vi "GetDefaultParams.vi"(8 "error in (no error)":errorcluster, 10 "Path":path, 11 "StandardFunction in":refnum<class "StandardFunction.lvclass">) -> (0 "error out":errorcluster, 3 "StandardFunction out":refnum<class "StandardFunction.lvclass">)   [LabVIEW 2018, in "Functions.lvlib" / "StandardFunction.lvclass"]
uses:
  StandardFunction.lvclass
  X:/Projects/NistPluggableModules/dev/NistPluggableModules/FGen/MemberClasses/FunctionBaseClass/FunctionBase.lvclass
  TypeDefs/StdWfrms.ctl
  TypeDefs/StdWfrm.ctl
  FunctionBaseClass/FunctionBase.lvclass/FunctionBase.ctl
  StandardFunction.lvclass/StandardFunction.ctl
  FunctionBaseClass/Accessors/Read FunctionIniFilePath.vi
  Accessors/Write StandardWfrms.vi
  FunctionBaseClass/FunctionBase.lvclass
  <vilib>/Utility/config.llb/NI_LVConfig.lvlib
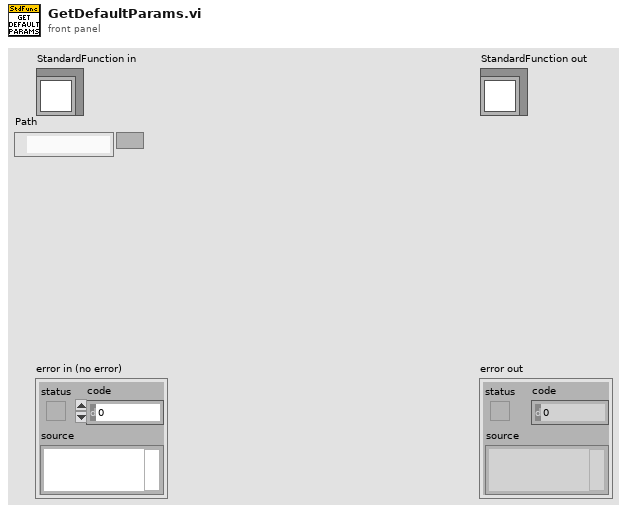
[diagram p1: front panel]
types:
  T1 = typedef "Functions.lvlib/StandardFunction.lvclass/StdWfrms.ctl" = cluster{"Count":u16, "StandardWfrm":T2[]}
  T2 = typedef "Functions.lvlib/StandardFunction.lvclass/StdWfrm.ctl" = cluster{"Amplitude":dbl, "DcOffset":dbl, "DutyCycle":dbl, "Frequency":dbl, "Phase":dbl, "Waveform":enum16{"Sine", "Square", "Triangle", "Ramp Up", "Ramp Down", "DC"}, "Handle":string}
  T3 = typedef "NI_LVConfig.lvlib/Config Data RefNum.ctl" = refnum<k1>
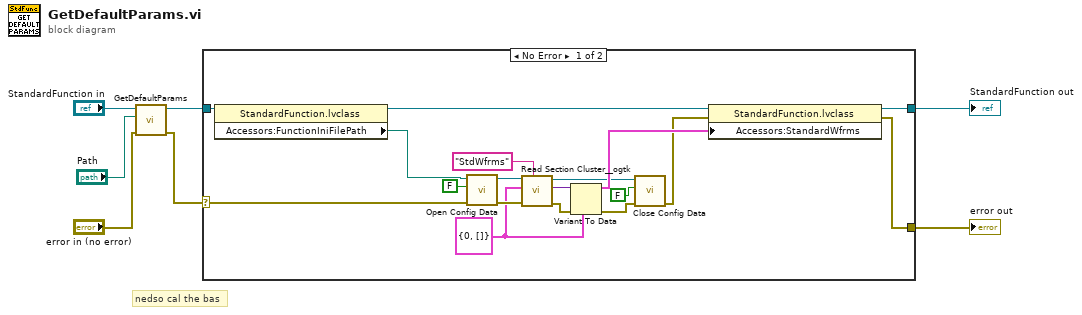
[diagram p0: block diagram]
diagram:
  # "nedso cal the bas"
  n1 = call-parent "GetDefaultParams.vi"("error in (no error)"="error in (no error)", "Path"="Path", "FunctionBase in"="StandardFunction in") -> ("error out"=w1:errorcluster, "FunctionBase out"=w4:refnum<class "StandardFunction.lvclass">)  [unwired: 7 in]
  n2 = case shown="No Error" w1 {
    selector: w1 -> [w21 w27]
    tunnel: [w16 w27] -> w7
    tunnel: [w18 w26] -> w6
    tunnel: w4 -> [w25 w26]
    frame No Error {
      w10 = T1 {"Count"=0, "StandardWfrm"=[]} ("StandardWfrms")
      n3 = property class="StandardFunction.lvclass"(reference=w25) -> (reference out=w9:refnum<class "StandardFunction.lvclass">, "Accessors:FunctionIniFilePath"=w8:path)  [unwired: 1 in, 1 out]
      n4 = call <vilib>:"Open Config Data.vi"("error in (no error)"=w21, "create file if necessary (T)"=FALSE, "configuration file path"=w8) -> ("error out"=w24:errorcluster, "refnum"=w23:T3)  [unwired: 6 in, 1 out]
      n5 = call <userlib>:"Read Section Cluster__ogtk.vi"("section (optional)"="StdWfrms", "error in (no error)"=w24, "Section Formatted Cluster Type"=w10, "refnum"=w23) -> ("error out"=w19:errorcluster, "Section Formatted Cluster"=w20:variant, "dup refnum"=w14:T3)  [unwired: 3 in, 2 out]
      n6 = Variant To Data(error in=w19, type=w10, Variant=w20) -> (data=w17:T1, error out=w13:errorcluster)
      n7 = call <vilib>:"Close Config Data.vi"("error in (no error)"=w13, "write file if changed (T)"=FALSE, "refnum"=w14) -> ("error out"=w12:errorcluster)  [unwired: 7 in, 1 out]
      n8 = property class="StandardFunction.lvclass"(reference=w9, error in=w12, "Accessors:StandardWfrms"=w17) -> (reference out=w18:refnum<class "StandardFunction.lvclass">, error out=w16:errorcluster)
    }
    frame Error {
    }
  }
  "error out" <- w7
  "StandardFunction out" <- w6
